vi "Control Mode.vi"(8 "error in (no error)":errorcluster, 9 "Timeout (30000 ms)":u32=30000, 10 "Control Mode (0:Local)":u16(ring) items=["Local", "Remote", "Remote with Lock"], 11 "VISA Resource Name":refnum<visa-resource-name>) -> (0 "error out":errorcluster, 3 "VISA Resource Out":refnum<visa-resource-name>)   [LabVIEW 2014, in "Agilent 34401.lvlib"]
doc: "Sets the multimeter for remote or local operation.\n\n<B>Note:</B>\n\n- This VI should only be run with an RS-232 serial interface.\n- A known issue with the instrument hardware causes the lock transition from Remote with Lock (RWL) to Remote (REM) to fail. This will vary based on instrument firmware version."
uses:
  <instrlib>/Agilent 34401/Agilent 34401.lvlib
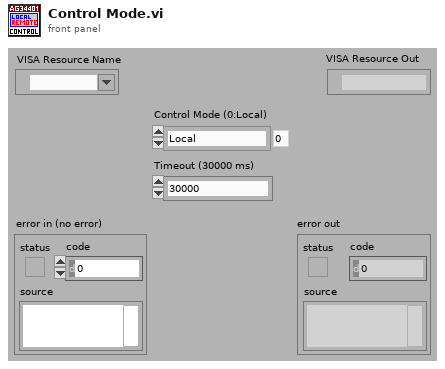
[diagram p1: front panel]
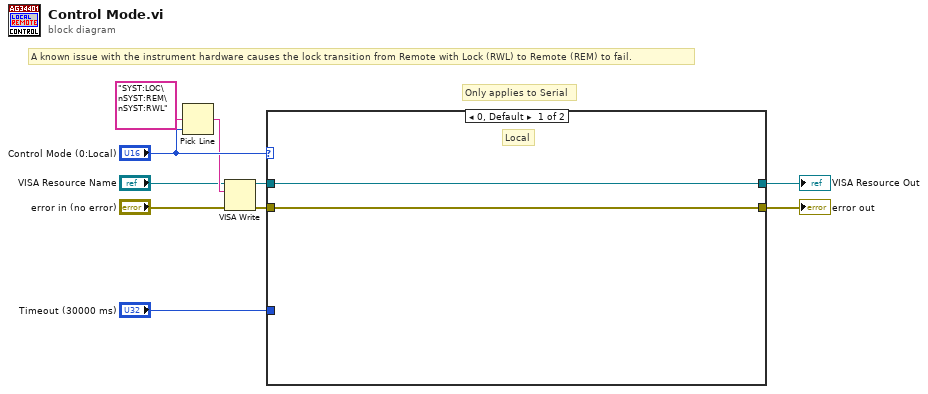
[diagram p0: block diagram]
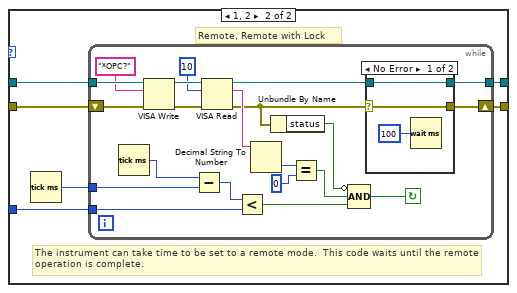
[diagram p2: hidden frame]
diagram:
  # "A known issue with the instrument hardware causes the lock transition from Remote with Lock (RWL) to Remote (REM) to fail."
  # "Only applies to Serial"
  n1 = Pick Line(multi-line string="SYST:LOC\nSYST:REM\nSYST:RWL", line index="Control Mode (0:Local)") -> (output string=w3:string)  [unwired: 1 in]
  n2 = VISA Write(VISA resource name="VISA Resource Name", write buffer=w3, error in (no error)="error in (no error)") -> (VISA resource name out=w6:refnum<visa-resource-name>, error out=w5:errorcluster)  [unwired: 1 out]
  n3 = case shown="0, Default" "Control Mode (0:Local)" {
    tunnel: w6 -> [w12 w18]
    tunnel: w5 -> [w11 w15]
    tunnel: [w12 w17] -> w8
    tunnel: [w11 w14] -> w7
    tunnel: "Timeout (30000 ms)" -> [_ w16]
    frame 0, Default {
      # "Local"
    }
    frame 1, 2 {
      # "The instrument can take time to be set to a remote mode.  This code waits until the remote operation is complete."
      # "Remote, Remote with Lock"
      n4 = Tick Count (ms)() -> (millisecond timer value=w13:u32)
      n5 = while {
        shift-left: w15 -> [w21]
        shift-right: [w25] -> w14
        tunnel: [w24] -> w17
        tunnel: w16 -> [w33]
        tunnel: w18 -> [w32]
        tunnel: w13 -> [w39]
        stop <- w37 continue-if-true
        n6 = Tick Count (ms)() -> (millisecond timer value=w19:u32)
        n7 = VISA Write(VISA resource name=w32, write buffer="*OPC?" ("write buffer (\"\")"), error in (no error)=w21) -> (VISA resource name out=w30:refnum<visa-resource-name>, error out=w29:errorcluster)  [unwired: 1 out]
        n8 = Subtract(x=w19, y=w39) -> (x-y=w34:u32)
        n9 = VISA Read(VISA resource name=w30, byte count=u32 10 ("byte count (0)"), error in (no error)=w29) -> (VISA resource name out=w23:refnum<visa-resource-name>, read buffer=w26:string, error out=w20:errorcluster)  [unwired: 1 out]
        n10 = Less?(x=w34, y=w33) -> (x < y?=w38:bool)
        n11 = Decimal String To Number(string=w26) -> (number=w27:i32)  [unwired: 2 in, 1 out]
        n12 = Unbundle By Name(w20) -> ("status"=w22:bool)
        n13 = Equal?(x=w27, y=0 ("*OPC Desired Response")) -> (x = y?=w35:bool)
        n14 = Compound Arithmetic op=AND(invert w22, w35, w38) -> (w37:bool)
        n15 = case shown="No Error" w20 {
          selector: w20 -> [w40 w43]
          tunnel: [w40 w43] -> w25
          tunnel: w23 -> [w41 w44]
          tunnel: [w41 w44] -> w24
          frame No Error {
            n16 = Wait (ms)(milliseconds to wait=u32 100) -> ()  [unwired: 1 out]
          }
          frame Error {
            # "Error\nNo Delay"
          }
        }
      }
    }
  }
  "error out" <- w7
  "VISA Resource Out" <- w8
